vi "Instantiate with Path.vi"(0 "LV Doc Path":path, 11 "error in (no error)":errorcluster) -> (4 "Document out":refnum<class "Document.lvclass">, 15 "error out":errorcluster)   [LabVIEW 2016, in "LV DEV.lvclass"]
uses:
  LV DEV.lvclass
  Document.lvclass
  D:/MDI Project/source code/Document/Document.lvclass
  D:/MDI Project/source code/Document/Child Classes/LV Doc/LV Doc.lvclass
  Document.lvclass/Document.ctl
  LV Doc.lvclass
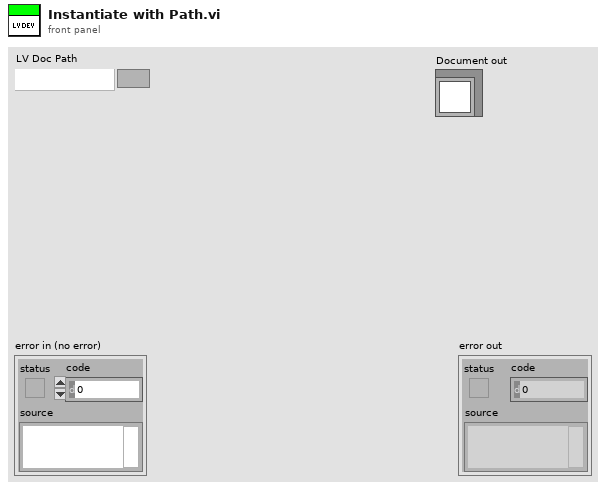
[diagram p1: front panel]
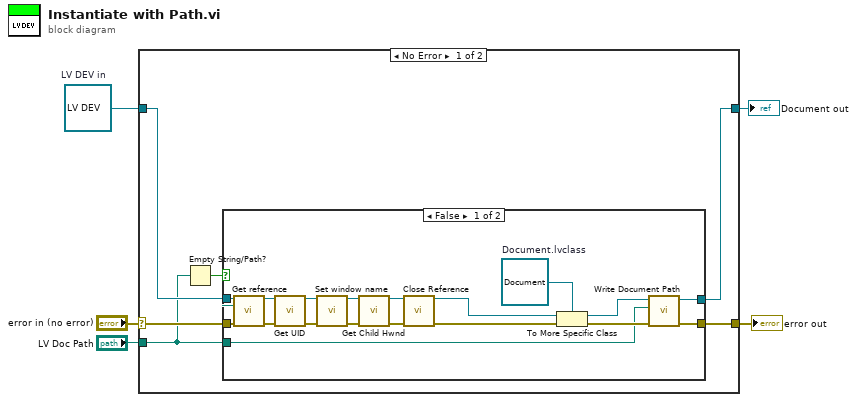
[diagram p0: block diagram]
diagram:
  w3 = refnum<class "LV DEV.lvclass"> refnum  # LV DEV in
  n1 = case shown="No Error" "error in (no error)" {
    selector: "error in (no error)" -> [w9 w32]
    tunnel: [w11 w32] -> w4
    tunnel: [w10 w31] -> w1
    tunnel: w3 -> [w8 w31]
    tunnel: "LV Doc Path" -> [w7 _]
    frame No Error {
      n2 = Empty String/Path?(string/path=w7) -> (empty?=w6:bool)
      n3 = case shown="False" w6 {
        tunnel: [w27 w30] -> w11
        tunnel: [w25 _] -> w10
        tunnel: w9 -> [w16 w30]
        tunnel: w8 -> [w13 _]
        tunnel: w7 -> [w12 _]
        frame False {
          w29 = refnum<class "Document.lvclass"> refnum  # Document.lvclass
          n4 = call "Get reference.vi"("LV Doc.lvclass"=w13, "Vi Path"=w12, "Error in"=w16) -> ("LV Doc.lvclass"=w14:refnum<class "LV DEV.lvclass">, "Error Out"=w15:errorcluster)  [unwired: 11 in]
          n5 = call "Get UID.vi"("LV Doc.lvclass"=w14, "error in (no error)"=w15) -> ("LV Doc.lvclass"=w17:refnum<class "LV DEV.lvclass">, "error out"=w18:errorcluster)  [unwired: 12 in]
          n6 = call "Set window name.vi"("LV Doc.lvclass"=w17, "error in (no error)"=w18) -> ("LV Doc.lvclass"=w19:refnum<class "LV DEV.lvclass">, "error out"=w20:errorcluster)  [unwired: 12 in]
          n7 = call "Get Child Hwnd.vi"("LV Doc.lvclass"=w19, "Error in"=w20) -> ("LV Doc.lvclass"=w21:refnum<class "LV DEV.lvclass">, "Error Out"=w22:errorcluster)  [unwired: 12 in]
          n8 = call "Close Reference.vi"("LV Doc in"=w21, "error in (no error)"=w22) -> ("LV Doc out"=w24:refnum<class "LV DEV.lvclass">, "error out"=w23:errorcluster)  [unwired: 12 in]
          n9 = To More Specific Class(target class=w29, reference=w24, error in=w23) -> (specific class reference=w28:refnum<class "Document.lvclass">, error out=w26:errorcluster)
          n10 = call "Write Document Path.vi"("error in (no error)"=w26, "Document Path"=w12, "Document in"=w28) -> ("error out"=w27:errorcluster, "Document out"=w25:refnum<class "Document.lvclass">)  [unwired: 7 in]
        }
        frame True {
        }
      }
    }
    frame Error {
    }
  }
  "error out" <- w4
  "Document out" <- w1
